vi "cam_Global.vi"() -> ()   [LabVIEW 2017, in "PlayNitrideCameraComponet1010_4.lvlib"]
uses:
  <userlib>/PlayNitrideCameraComponet1010_4/PlayNitrideCameraComponet1010_4.lvlib
panel:
  in  "crop_suffix":string
  out "Global Rectangle":i32[](array[numeric])
  in  "img_suffix":string
  in  "manual_suffix":string
  in  "failure_suffix":string
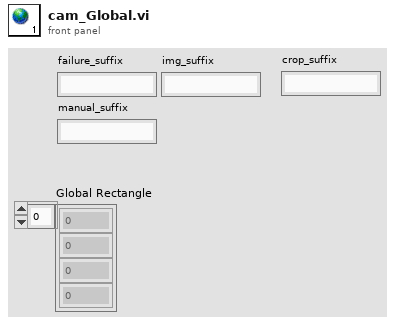
[diagram p1: front panel]
diagram:
